vi "数据补发判定有限循环.vi"(8 "错误输入（无错误）":errorcluster, 9 "数据输入":string, 10 "QN":string, 11 "数据发送通道":enum16{"TCP", "VISA"}(ring)) -> (3 "error out":errorcluster)   [LabVIEW 2016, in "数据传输系统-02.lvlib"]
uses:
  <vilib>/ptbypt/NI_PtbyPt.lvlib
panel:
  out "重发次数":dbl
  out "x+1":u32
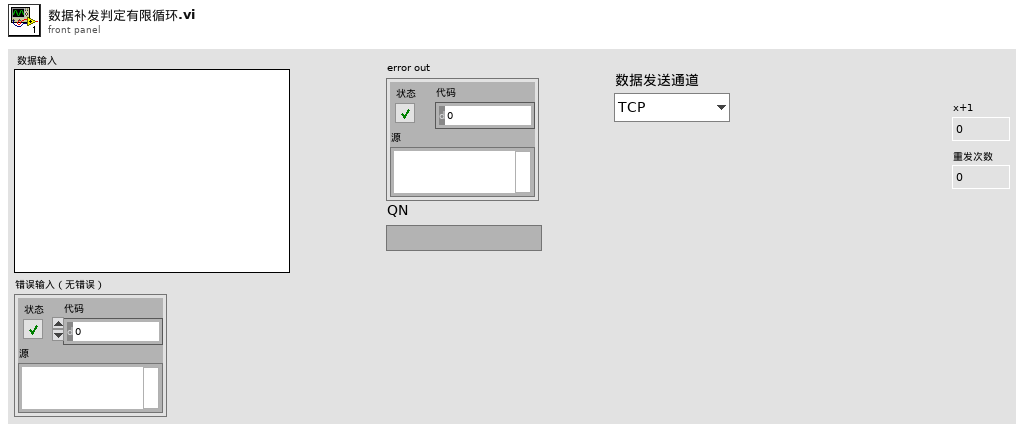
[diagram p1: front panel]
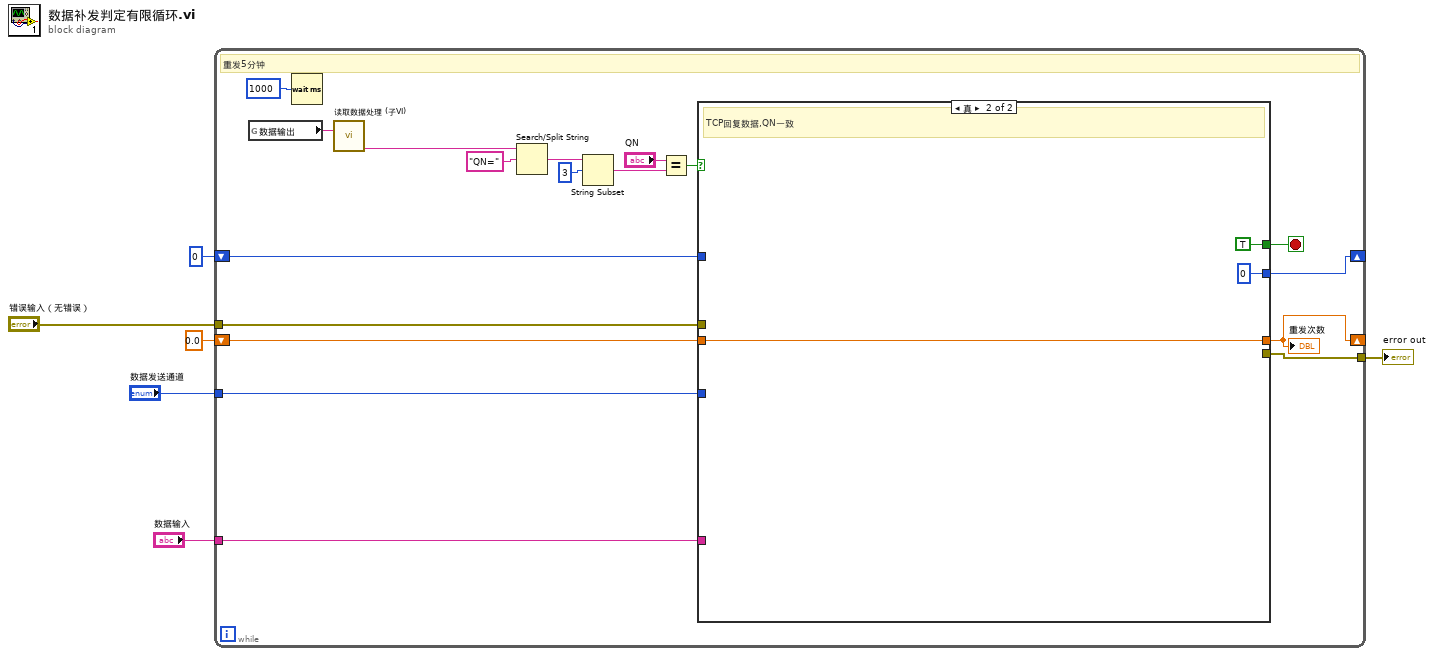
[diagram p0: block diagram]
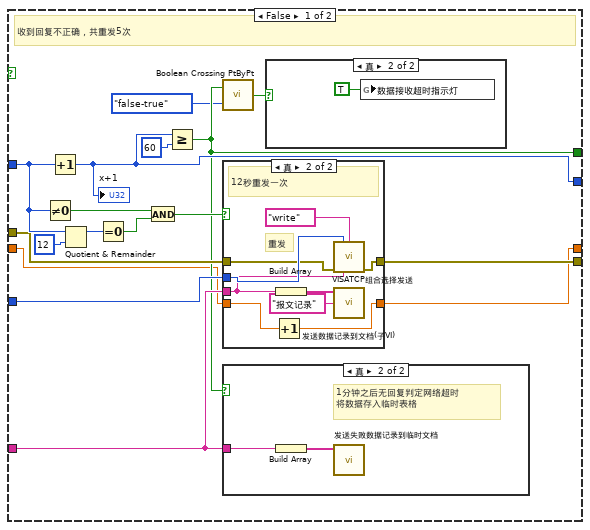
[diagram p2: hidden frame]
diagram:
  n1 = while {
    shift-right: [w22] -> _
    shift-left: u32 0 ("等待时间（毫秒）") -> [w23]
    tunnel: "数据发送通道" -> [w19]
    tunnel: [w18] -> w5
    tunnel: "数据输入" -> [w17]
    tunnel: "错误输入（无错误）" -> [w16]
    shift-right: [w7] -> _
    shift-left: 0.0 ("重发次数") -> [w8]
    stop <- w21 stop-if-true
    # "重发5分钟"
    n2 = global read "全局1.vi" "数据输出"() -> (w11:string)
    n3 = Wait (ms)(milliseconds to wait=u32 1000 ("等待时间（毫秒）")) -> ()  [unwired: 1 out]
    n4 = call "读取数据处理 (子VI).vi"("data out"=w11) -> ("时间QN"=w15:string)  [unwired: 8 in, 6 out]
    n5 = Search/Split String(string=w15, search string/char (-)="QN=" ("搜索字符串/字符(-)")) -> (match + rest of string=w14:string)  [unwired: 1 in, 2 out]
    n6 = String Subset(string=w14, offset (0)=3 ("偏移量(0)")) -> (substring=w10:string)  [unwired: 1 in]
    n7 = Equal?(x="QN", y=w10) -> (x = y?=w20:bool)
    n8 = case shown="真" w20 {
      tunnel: w23 -> [w35 _]
      tunnel: [w40 u32 0] -> w22
      tunnel: [w29 TRUE] -> w21
      tunnel: w19 -> [w33 _]
      tunnel: [w32 _] -> w18
      tunnel: w17 -> [w30 _]
      tunnel: w16 -> [w31 _]
      tunnel: w8 -> [w26 w56]
      tunnel: [w25 w56] -> w7
      frame False {
        # "收到回复不正确，共重发5次"
        n9 = Not Equal To 0?(x=w35) -> (x != 0?=w34:bool)
        n10 = Increment(x=w35) -> (x+1=w40:u32)
        "x+1" <- w40
        n11 = Quotient & Remainder(x=w35, y=u32 12) -> (x-y*floor(x/y)=w38:u32)  [unwired: 1 out]
        n12 = Equal To 0?(x=w38) -> (x = 0?=w37:bool)
        n13 = And(x=w34, y=w37) -> (x .and. y?=w36:bool)
        n14 = Greater Or Equal?(x=w40, y=u32 60) -> (x >= y?=w29:bool)
        n15 = call <vilib>:"Boolean Crossing PtByPt.vi"("direction"=enum16{"either", "false-true", "true-false"}."false-true", "input"=w29) -> ("crossing"=w27:bool)  [unwired: 1 in]
        n16 = case shown="真" w36 {
          tunnel: w33 -> [_ w54]
          tunnel: [w46 w50] -> w32
          tunnel: w30 -> [_ w52]
          tunnel: w31 -> [w46 w51]
          tunnel: w26 -> [w45 w49]
          tunnel: [w45 w48] -> w25
          frame False {
          }
          frame True {
            # "重发"
            # "12秒重发一次"
            n17 = Increment(x=w49) -> (x+1=w48:dbl)
            n18 = Build Array(w52) -> (w55:string[])
            n19 = call "VISATCP组合选择发送.vi"("数据发送通道"=w54, "命令"="write", "error in (no error)"=w51, "写入缓冲区"=w52) -> ("错误输出"=w50:errorcluster)  [unwired: 8 in, 3 out]
            n20 = call "发送数据记录到文档(子VI).vi"("字符串"="报文记录", "数组"=w55) -> ()  [unwired: 8 in, 1 out]
          }
        }
        n21 = case shown="真" w29 {
          tunnel: w30 -> [_ w43]
          frame False {
          }
          frame True {
            # "1分钟之后无回复判定网络超时\n将数据存入临时表格"
            n22 = Build Array(w43) -> (w44:string[])
            n23 = call "发送失败数据记录到临时文档.vi"("数组"=w44) -> ()  [unwired: 9 in, 1 out]
          }
        }
        n24 = case shown="真" w27 {
          frame False {
          }
          frame True {
            n25 = global write "全局 数据发送重叠.vi" "数据接收超时指示灯"(TRUE ("数据接收超时指示灯")) -> ()
          }
        }
      }
      frame True {
        # "TCP回复数据,QN一致"
      }
    }
    "重发次数" <- w7
  }
  "error out" <- w5
